vi "Set Front Panel Custom Image Size Cluster Control.vi"(8 "error in (no error)":errorcluster, 9 "Enable/Disable":bool, 10 "Init":bool, 11 "Cluster Ref In":refnum<vi>) -> (0 "error IO":errorcluster)   [LabVIEW 2018]
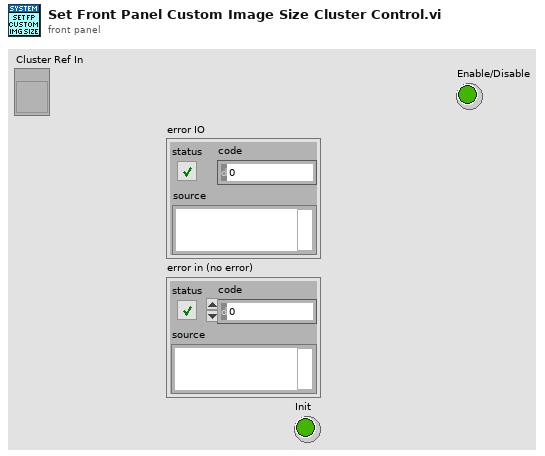
[diagram p1: front panel]
types:
  T1 = enum8{"Enabled", "Disabled", "Disabled and Grayed Out"}
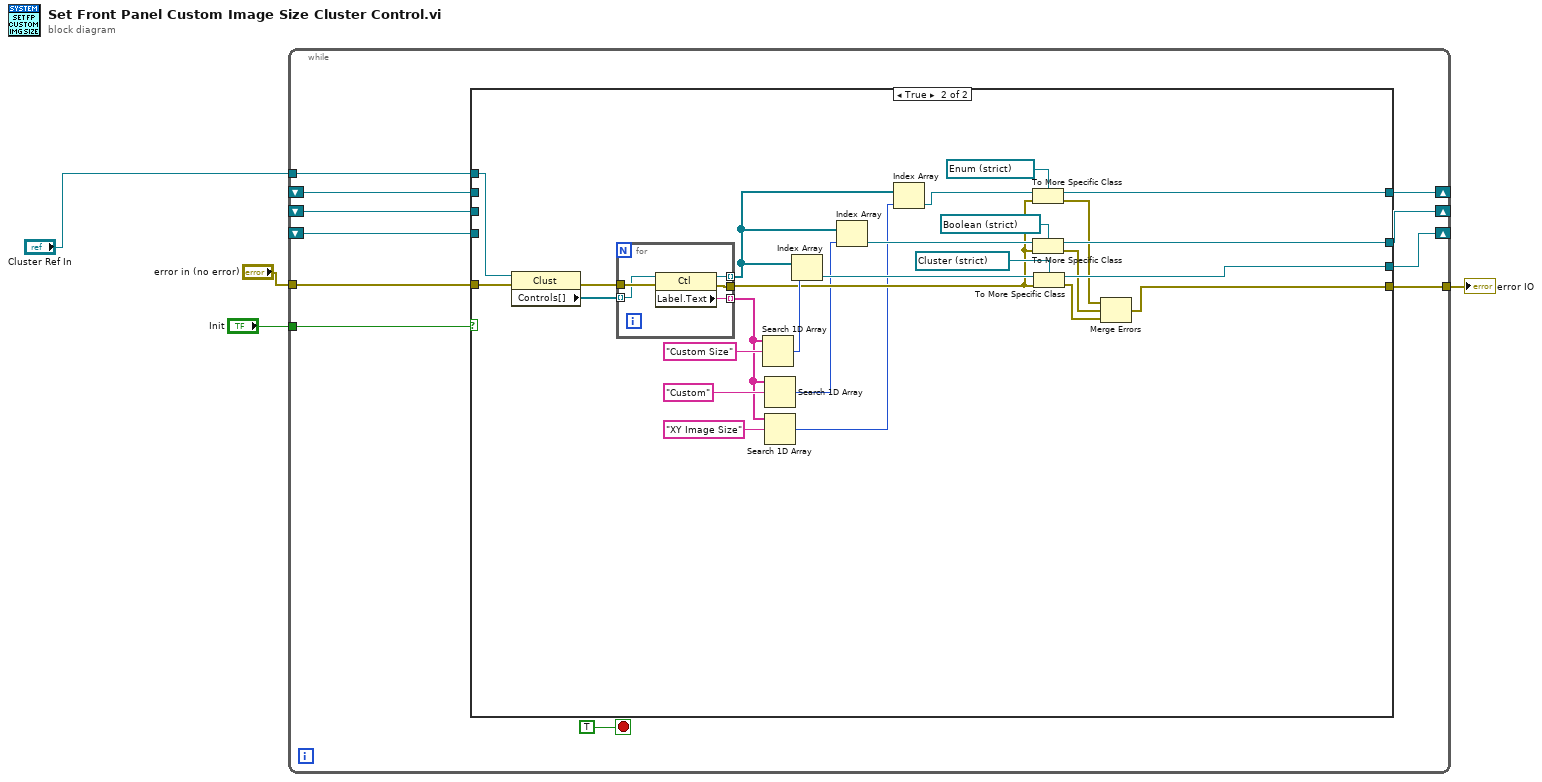
[diagram p0: block diagram]
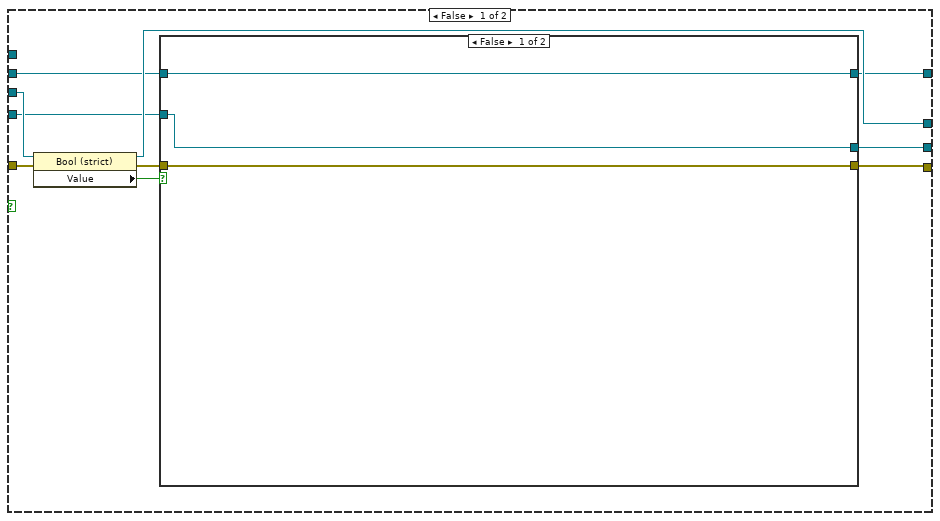
[diagram p2: hidden frame]
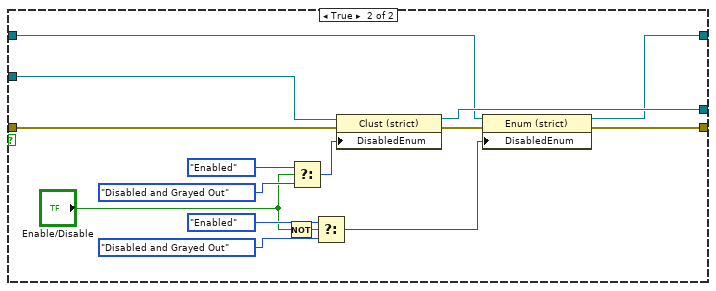
[diagram p3: hidden frame]
diagram:
  n1 = while {
    tunnel: "Cluster Ref In" -> [w15]
    tunnel: [w12] -> w4
    tunnel: "error in (no error)" -> [w11]
    shift-right: [w13] -> _
    shift-left: _ -> [w10]
    tunnel: "Init" -> [w9]
    shift-right: [w8] -> _
    shift-left: _ -> [w7]
    shift-right: [w6] -> _
    shift-left: _ -> [w5]
    stop <- TRUE stop-if-true
    n2 = case shown="True" w9 {
      tunnel: w15 -> [_ w69]
      tunnel: [w22 w59] -> w13
      tunnel: [w19 w56] -> w12
      tunnel: w11 -> [w25 w66]
      tunnel: w10 -> [w20 _]
      tunnel: [w21 w60] -> w8
      tunnel: w7 -> [w23 _]
      tunnel: [w17 w51] -> w6
      tunnel: w5 -> [w18 _]
      frame False {
        n3 = property class="Bool (strict)"(reference=w23, error in=w25) -> (reference out=w21:refnum<vi>, error out=w24:errorcluster, "Value"=w16:bool)
        n4 = case shown="False" w16 {
          tunnel: w24 -> [w28 w43]
          tunnel: [w26 w41] -> w22
          tunnel: w20 -> [w26 w40]
          tunnel: [w28 w36] -> w19
          tunnel: w18 -> [w27 w35]
          tunnel: [w27 w34] -> w17
          frame False {
          }
          frame True {
            n5 = Not(x="Enable/Disable") -> (.not. x?=w31:bool)
            n6 = Select(t=T1."Enabled" ("Disabled"), s="Enable/Disable", f=T1."Disabled and Grayed Out" ("Disabled")) -> (s? t:f=w37:T1)
            n7 = Select(t=T1."Enabled" ("Disabled"), s=w31, f=T1."Disabled and Grayed Out" ("Disabled")) -> (s? t:f=w30:T1)
            n8 = property class="Clust (strict)"(reference=w40, error in=w43, "DisabledEnum"=w37) -> (reference out=w41:refnum<vi>, error out=w42:errorcluster)
            n9 = property class="Enum (strict)"(reference=w35, error in=w42, "DisabledEnum"=w30) -> (reference out=w34:refnum<vi>, error out=w36:errorcluster)
          }
        }
      }
      frame True {
        n10 = property class="Clust"(reference=w69, error in=w66) -> (error out=w67:errorcluster, "Controls[]"=w68:refnum<vi>[])  [unwired: 1 out]
        n11 = for {
          tunnel: w68 -> [w73] mode=indexing
          tunnel: w67 -> [w74]
          tunnel: [w72] -> w46 mode=indexing
          tunnel: [w71] -> w49 mode=indexing
          tunnel: [w70] -> w50
          n12 = property class="Ctl"(reference=w73, error in=w74) -> (reference out=w71:refnum<vi>, error out=w70:errorcluster, "Label.Text"=w72:string)
        }
        n13 = Search 1D Array(1D array=w46, element="Custom Size") -> (index of element=w63:i32)  [unwired: 1 in]
        n14 = Search 1D Array(1D array=w46, element="Custom") -> (index of element=w47:i32)  [unwired: 1 in]
        n15 = Search 1D Array(1D array=w46, element="XY Image Size") -> (index of element=w44:i32)  [unwired: 1 in]
        n16 = Index Array(array=w49, index=w63) -> (element=w64:refnum<vi>)
        n17 = Index Array(array=w49, index=w47) -> (element=w61:refnum<vi>)
        n18 = Index Array(array=w49, index=w44) -> (element=w48:refnum<vi>)
        n19 = To More Specific Class(target class=refnum<vi> refnum ("XY Image Size"), reference=w48, error in=w50) -> (specific class reference=w51:refnum<vi>, error out=w52:errorcluster)
        n20 = To More Specific Class(target class=refnum<vi> refnum ("Boolean"), reference=w61, error in=w50) -> (specific class reference=w60:refnum<vi>, error out=w57:errorcluster)
        n21 = To More Specific Class(target class=refnum<vi> refnum ("Custom Size"), reference=w64, error in=w50) -> (specific class reference=w59:refnum<vi>, error out=w58:errorcluster)
        n22 = Merge Errors(w52, w57, w58) -> (w56:errorcluster)
      }
    }
  }
  "error IO" <- w4
